vi "HypervisorAdd.vi"(6 "StopHpvsr":bool, 8 "ErrorIn":errorcluster, 9 "Data":variant, 10 "ItemName":string, 11 "QIn":refnum<queue>) -> (0 "ErrorOut":errorcluster, 3 "QOut":refnum<queue>)   [LabVIEW 2018]
doc: "Add a new item to the Hypervisor event queue.\n\nInput a descriptor for the event, whether to issue Stop to the Hypervisor Write Loop and any data to be logged with the the event. This VI adds a timestamp to the aforemented sevent.\n\nCopyright © 2019 Epimedia, Inc. All Rights Reserved.\n\nThe Epimedia Application Library is Copyright © 2009-2017 Epimedia, Inc. \nAll Rights Reserved. Used under license."
uses:
  Queue/HyperVisor.ctl
panel:
  # "Copyright © 2019 Epimedia, Inc. All Rights Reserved.\n\nThe Epimedia Application Library is Copyright © 2009-2017 Epimedia, Inc. \nAll Rights Reserved. Used under license."
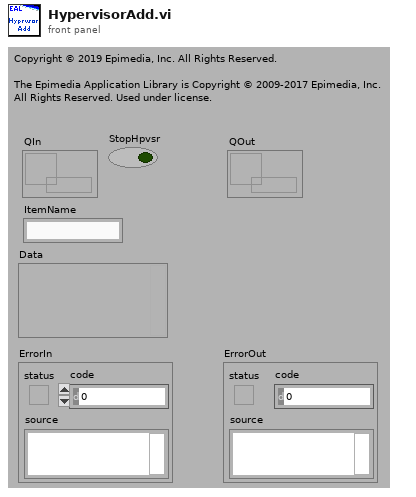
[diagram p1: front panel]
types:
  T1 = typedef "HyperVisor.ctl" = cluster{"TimeOut":dbl, string, "Data":variant, "StopHpvsr":bool}
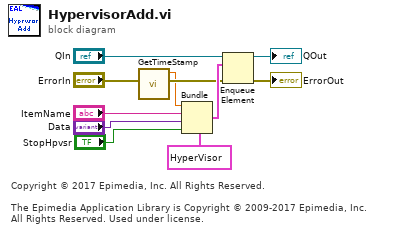
[diagram p0: block diagram]
diagram:
  # "Copyright © 2017 Epimedia, Inc. All Rights Reserved.\n\nThe Epimedia Application Library is Copyright © 2009-2017 Epimedia, Inc. \nAll Rights Reserved. Used under license."
  n1 = call "GetTimeStamp.vi"("ErrorIn"="ErrorIn") -> ("ErrorOut"=w2:errorcluster, "TimeOut"=w1:dbl)  [unwired: 3 in, 6 out]
  n2 = Bundle(cluster=T1 {"TimeOut"=0.0, "", "Data"=variant, "StopHpvsr"=FALSE} ("HprVsr"), "TimeOut"=w1, "ItemName", "Data"="Data", "StopHpvsr"="StopHpvsr") -> (w11:T1)
  n3 = Enqueue Element(queue="QIn", element=w11, error in (no error)=w2) -> (queue out=→"QOut":refnum<queue>, error out=→"ErrorOut":errorcluster)  [unwired: 1 in, 1 out]
